vi "_CSTK_Button_Icon_ResizeButtonSize.vi"(7 "XControl:容器边界":T1 caption="边界", 9 "NewBnds":T2, 10 "OldBnds":T2, 11 "Display State 输入":T3 caption="Display State Out") -> (3 "Display State 输出":T3 caption="Display State Out")   [LabVIEW 2015, in "CSTK_Button_Icon.xctl"]
uses:
  CSTK_Button_Icon.xctl
  CSTK_Button_Icon_Status.ctl
  TypeDefinitions/_CSTK_Button_Icon_ButtonSize.ctl
  <vilib>/Utility/miscctls.llb/LVBoundsTypeDef.ctl
  TypeDefinitions/_CSTK_Button_Icon_LogoImage.ctl
  <vilib>/picture/picture.llb/imagedata.ctl
  TypeDefinitions/_CSTK_Button_Icon_LogoProperties.ctl
  TypeDefinitions/_CSTK_Button_Icon_LogoProperties_Data.ctl
  TypeDefinitions/_CSTK_Button_Icon_TextString.ctl
  TypeDefinitions/_CSTK_Button_Icon_TextProperties.ctl
  TypeDefinitions/_CSTK_Button_Icon_TextProperties_Data.ctl
  TypeDefinitions/_CSTK_Button_Icon_TextProperties_FontStyle.ctl
  TypeDefinitions/_CSTK_Button_Icon_BGColor.ctl
  TypeDefinitions/_CSTK_Button_Icon_BorderColor.ctl
  TypeDefinitions/_CSTK_Button_Icon_BorderProperties.ctl
  TypeDefinitions/_CSTK_Button_Icon_BorderProperties_Data.ctl
  TypeDefinitions/_CSTK_Button_Icon_CurrentBGImage.ctl
  TypeDefinitions/_CSTK_Button_Icon_DrawAreaSize.ctl
  TypeDefinitions/_CSTK_Button_Icon_TextStartOffset.ctl
  <vilib>/Utility/miscctls.llb/LVRectTypeDef.ctl
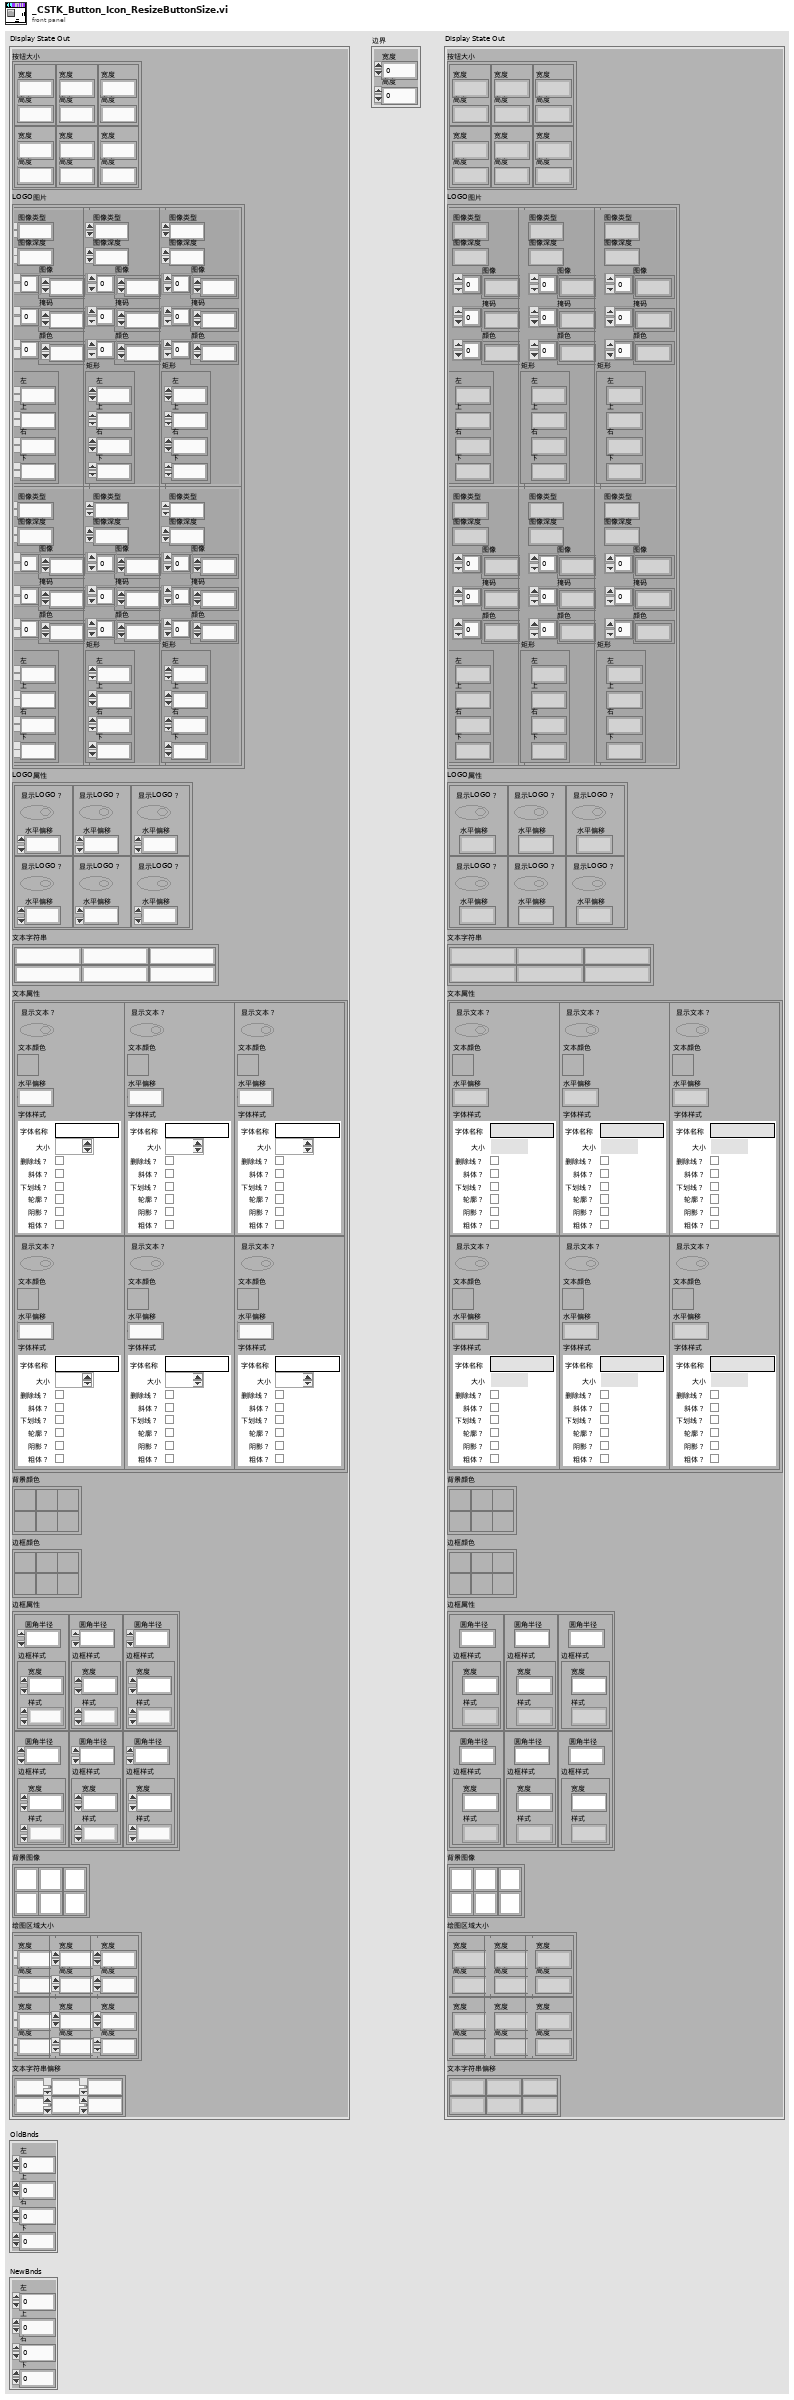
[diagram p1: front panel]
types:
  T1 = typedef "LVBoundsTypeDef.ctl" = cluster{"Width":u32, "Height":u32}
  T2 = typedef "LVRectTypeDef.ctl" = cluster{"Left":i16, "Top":i16, "Right":i16, "Bottom":i16}
  T3 = typedef "CSTK_Button_Icon.xctl/CSTK_Button_Icon_Status.ctl" = cluster{"ButtonSize":T4, "Logo Image":T5, "Logo Properties":T7, "Text String":T9, "Text Properties":T10, "BG Color":T13, "Border Color":T14, "Border Properties":T15, "Current BG Image":T17, "DrawAreaSize":T18, "Text String Offset":T19}
  T4 = typedef "CSTK_Button_Icon.xctl/_CSTK_Button_Icon_ButtonSize.ctl" = cluster{"False":T1, "True":T1, "True to False":T1, "False to True":T1, "Hover in False":T1, "Hover in True":T1}
  T5 = typedef "CSTK_Button_Icon.xctl/_CSTK_Button_Icon_LogoImage.ctl" = cluster{"False":T6, "True":T6, "True to False":T6, "False to True":T6, "Hover in False":T6, "Hover in True":T6}
  T6 = typedef "imagedata.ctl" = cluster{"image type":i32, "image depth":i32, "image":u8[], "mask":u8[], "colors":u32[], "Rectangle":cluster{"left":i16, "top":i16, "right":i16, "bottom":i16}}
  T7 = typedef "CSTK_Button_Icon.xctl/_CSTK_Button_Icon_LogoProperties.ctl" = cluster{"False":T8, "True":T8, "True to False":T8, "False to True":T8, "Hover in False":T8, "Hover in True":T8}
  T8 = typedef "CSTK_Button_Icon.xctl/_CSTK_Button_Icon_LogoProperties_Data.ctl" = cluster{"Display Logo?":bool, "Horizontal Offset":i16}
  T9 = typedef "CSTK_Button_Icon.xctl/_CSTK_Button_Icon_TextString.ctl" = cluster{"False":string, "True":string, "True to False":string, "False to True":string, "Hover in False":string, "Hover in True":string}
  T10 = typedef "CSTK_Button_Icon.xctl/_CSTK_Button_Icon_TextProperties.ctl" = cluster{"False":T11, "True":T11, "True to False":T11, "False to True":T11, "Hover in False":T11, "Hover in True":T11}
  T11 = typedef "CSTK_Button_Icon.xctl/_CSTK_Button_Icon_TextProperties_Data.ctl" = cluster{"Display Text?":bool, "Text Color":u32, "Horizontal Offset":i16, "Font Style":T12}
  T12 = typedef "CSTK_Button_Icon.xctl/_CSTK_Button_Icon_TextProperties_FontStyle.ctl" = cluster{"Font Name":string, "Size":i16, "Strikeout?":bool, "Italic?":bool, "Underline?":bool, "Outline?":bool, "Shadow?":bool, "Bold?":bool}
  T13 = typedef "CSTK_Button_Icon.xctl/_CSTK_Button_Icon_BGColor.ctl" = cluster{"False":u32, "True":u32, "True to False":u32, "False to True":u32, "Hover in False":u32, "Hover in True":u32}
  T14 = typedef "CSTK_Button_Icon.xctl/_CSTK_Button_Icon_BorderColor.ctl" = cluster{"False":u32, "True":u32, "True to False":u32, "False to True":u32, "Hover in False":u32, "Hover in True":u32}
  T15 = typedef "CSTK_Button_Icon.xctl/_CSTK_Button_Icon_BorderProperties.ctl" = cluster{"False":T16, "True":T16, "True to False":T16, "False to True":T16, "Hover in False":T16, "Hover in True":T16}
  T16 = typedef "CSTK_Button_Icon.xctl/_CSTK_Button_Icon_BorderProperties_Data.ctl" = cluster{"Radius":i16, "Border Style":cluster{"Width":u16, "Style":enum32{"Solid", "Dash", "Dot", "DashDot", "DashDotDot"}}}
  T17 = typedef "CSTK_Button_Icon.xctl/_CSTK_Button_Icon_CurrentBGImage.ctl" = cluster{"False":picture, "True":picture, "True to False":picture, "False to True":picture, "Hover in False":picture, "Hover in True":picture}
  T18 = typedef "CSTK_Button_Icon.xctl/_CSTK_Button_Icon_DrawAreaSize.ctl" = cluster{"False":T1, "True":T1, "True to False":T1, "False to True":T1, "Hover in False":T1, "Hover in True":T1}
  T19 = typedef "CSTK_Button_Icon.xctl/_CSTK_Button_Icon_TextStartOffset.ctl" = cluster{"False":i32, "True":i32, "True to False":i32, "False to True":i32, "Hover in False":i32, "Hover in True":i32}
  T20 = cluster{"[0]":T1, "[1]":T1, "[2]":T1, "[3]":T1, "[4]":T1, "[5]":T1}
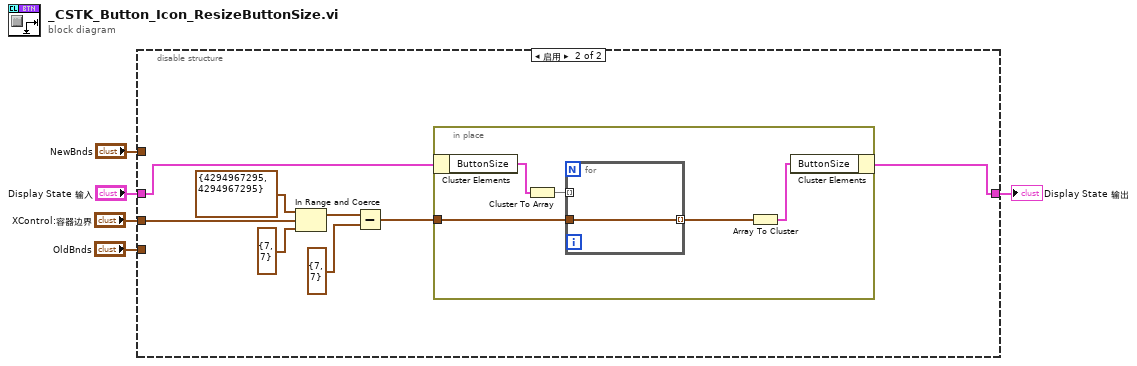
[diagram p0: block diagram]
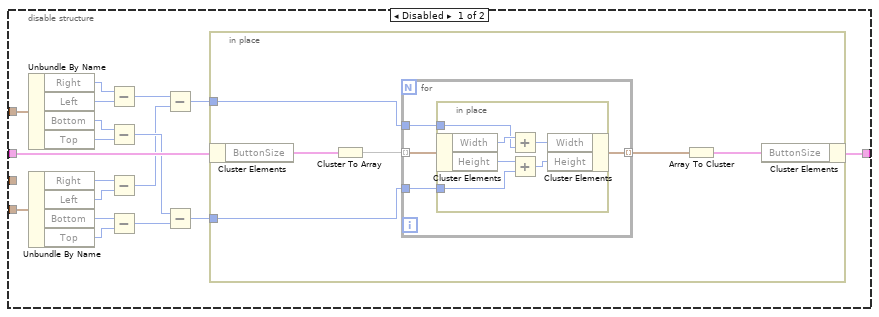
[diagram p2: hidden frame]
diagram:
  n1 = disable-structure shown="启用" {
    disable-tunnel: "OldBnds" -> [w23 _]
    disable-tunnel: "NewBnds" -> [w22 _]
    disable-tunnel: "Display State 输入" -> [w21 w42]
    disable-tunnel: [w20 w41] -> w2
    disable-tunnel: "XControl:容器边界" -> [_ w46]
    frame Disabled {
      n2 = Unbundle By Name(w22) -> ("Right"=w7:i16, "Left"=w6:i16, "Bottom"=w8:i16, "Top"=w9:i16)
      n3 = Unbundle By Name(w23) -> ("Right"=w11:i16, "Left"=w10:i16, "Bottom"=w12:i16, "Top"=w13:i16)
      n4 = Subtract(x=w7, y=w6) -> (x-y=w14:i16)
      n5 = Subtract(x=w8, y=w9) -> (x-y=w17:i16)
      n6 = Subtract(x=w11, y=w10) -> (x-y=w15:i16)
      n7 = Subtract(x=w12, y=w13) -> (x-y=w16:i16)
      n8 = Subtract(x=w14, y=w15) -> (x-y=w18:i16)
      n9 = Subtract(x=w17, y=w16) -> (x-y=w19:i16)
      n10 = in-place {
        in-place-border: w18 -> [w25]
        in-place-border: w19 -> [w24]
        n11 = in-place-cluster #1(w21) -> ("ButtonSize"=w29:T4)
        n12 = Cluster To Array(cluster=w29) -> (array=w28:T1[])
        n13 = for {
          tunnel: w28 -> [w33] mode=indexing
          tunnel: [w32] -> w27 mode=indexing
          tunnel: w25 -> [w31]
          tunnel: w24 -> [w30]
          n14 = in-place {
            in-place-border: w31 -> [w38]
            in-place-border: w30 -> [w35]
            n15 = in-place-cluster #2(w33) -> ("Width"=w39:u32, "Height"=w36:u32)
            n16 = Add(x=w39, y=w38) -> (x+y=w37:u32)
            n17 = Add(x=w36, y=w35) -> (x+y=w34:u32)
            n18 = in-place-cluster #2("Width"=w37, "Height"=w34) -> (w32:T1)
          }
        }
        n19 = Array To Cluster(array=w27) -> (cluster=w26:T20)
        n20 = in-place-cluster #1("ButtonSize"=w26) -> (w20:T3)
      }
    }
    frame Enabled {
      n21 = In Range and Coerce(upper limit=T1 {"Width"=4294967295, "Height"=4294967295} ("上限"), x=w46, lower limit=T1 {"Width"=7, "Height"=7} ("下限")) -> (coerced(x)=w43:T1)  [unwired: 1 out]
      n22 = Subtract(x=w43, y=T1 {"Width"=7, "Height"=7}) -> (x-y=w40:T1)
      n23 = in-place {
        in-place-border: w40 -> [w48]
        n24 = in-place-cluster #3(w42) -> ("ButtonSize"=w52:T4)
        n25 = Cluster To Array(cluster=w52) -> (array=w51:T1[])
        n26 = for {
          tunnel: w51 -> [_] mode=indexing
          tunnel: [w53] -> w50 mode=indexing
          tunnel: w48 -> [w53]
        }
        n27 = Array To Cluster(array=w50) -> (cluster=w49:T20)
        n28 = in-place-cluster #3("ButtonSize"=w49) -> (w41:T3)
      }
    }
  }
  "Display State 输出" <- w2
